vi "Get Child Name[].vi"(8 "error in (no error)":errorcluster, 11 "LV Doc.lvclass":refnum<class "LV Doc.lvclass">) -> (0 "error out":errorcluster, 2 "Array":string[](array[string]), 3 "LV Doc.lvclass":refnum<class "LV Doc.lvclass">)   [LabVIEW 2016, in "LV Doc.lvclass"]
doc: "Get all Child Window Hwnd."
uses:
  LV Doc.lvclass
  LV Doc.lvclass/LV Doc.ctl
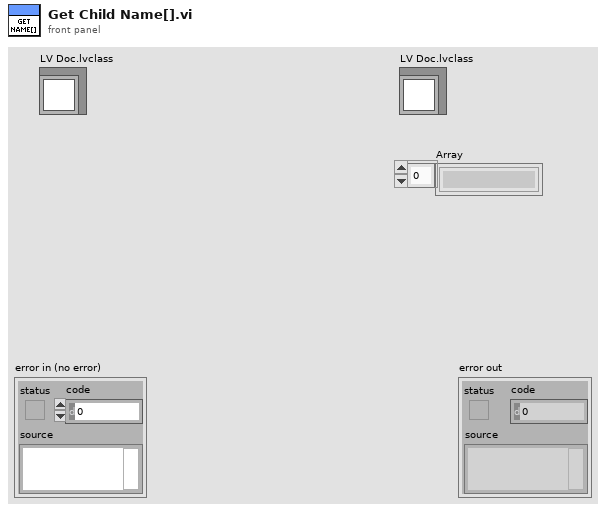
[diagram p1: front panel]
types:
  T1 = typedef "LV MDI.lvclass/Child Window Data.ctl" = cluster{"Child hWnd":u32, "UID":string, "vi reference":refnum<vi>, "Name":string}
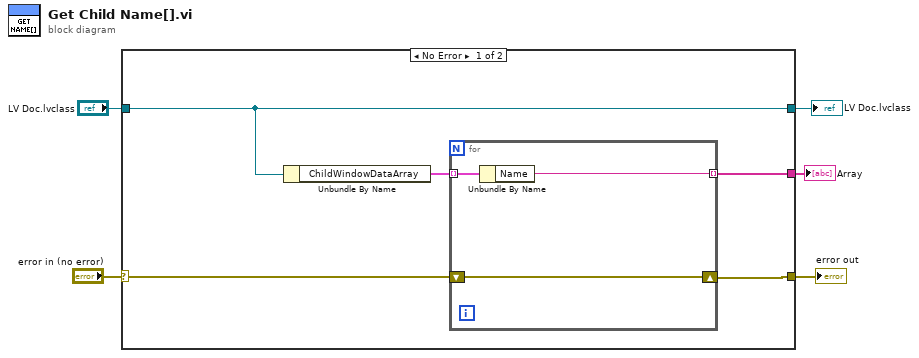
[diagram p0: block diagram]
diagram:
  n1 = case shown="No Error" "error in (no error)" {
    selector: "error in (no error)" -> [w9 w15]
    tunnel: [w8 w15] -> w4
    tunnel: [w10 w14] -> w1
    tunnel: "LV Doc.lvclass" -> [w10 w14]
    tunnel: [w6 _] -> w3
    frame No Error {
      n2 = Unbundle By Name(w10) -> ("ChildWindowDataArray"=w7:T1[])
      n3 = for {
        shift-right: [w13] -> w8
        shift-left: w9 -> [w13]
        tunnel: w7 -> [w12] mode=indexing
        tunnel: [w11] -> w6 mode=indexing
        n4 = Unbundle By Name(w12) -> ("Name"=w11:string)
      }
    }
    frame Error {
    }
  }
  "error out" <- w4
  "Array" <- w3
  "LV Doc.lvclass" <- w1
